vi "pad with zeroes - three string.vi"(3 "String 3 input":string, 4 "String 2 input":string, 5 "String 1 input":string) -> (0 "String 3 output":string, 1 "String 2 output":string, 2 "String 1 output":string)   [LabVIEW 2012]
doc: "This takes three strings (presumably of 0s and 1s), and pads the shorter two with zeroes so that they have the same length as the longer one."
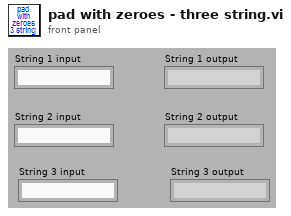
[diagram p1: front panel]
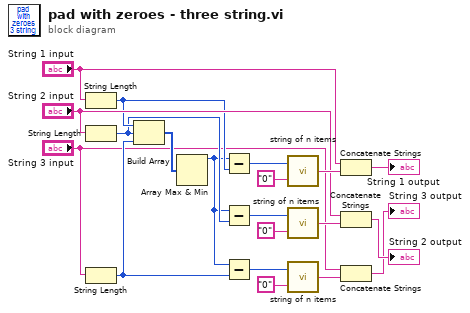
[diagram p0: block diagram]
diagram:
  n1 = String Length(string="String 1 input") -> (length=w9:i32)
  n2 = String Length(string="String 2 input") -> (length=w8:i32)
  n3 = String Length(string="String 3 input") -> (length=w6:i32)
  n4 = Build Array(w9, w8, w6) -> (w10:i32[])
  n5 = Array Max & Min(array=w10) -> (max value=w7:i32)  [unwired: 3 out]
  n6 = Subtract(x=w7, y=w9) -> (x-y=w14:i32)
  n7 = Subtract(x=w7, y=w8) -> (x-y=w16:i32)
  n8 = Subtract(x=w7, y=w6) -> (x-y=w4:i32)
  n9 = call "string of n items.vi"("string"="0", "Numeric"=w14) -> ("String"=w17:string)
  n10 = call "string of n items.vi"("string"="0", "Numeric"=w16) -> ("String"=w18:string)
  n11 = call "string of n items.vi"("string"="0", "Numeric"=w4) -> ("String"=w3:string)
  n12 = Concatenate Strings("String 1 input", w17) -> (→"String 1 output":string)
  n13 = Concatenate Strings("String 2 input", w18) -> (→"String 2 output":string)
  n14 = Concatenate Strings("String 3 input", w3) -> (→"String 3 output":string)
